vi "F-Truncat-IBRF.vi"() -> ()   [LabVIEW 2014]
doc: "Use this template to build a VI to use as a subVI."
uses:
  <vilib>/vision/NI_Vision_Development_Module.lvlib
panel:
  out "|F(u,v)H(u,v)|":T1(plugin-control)
  out "g(x,y)":T1(plugin-control)
  out "IF(u,v)I":T1(plugin-control)
  out "f(x,y)":T1(plugin-control)
  # ":: MVi Framework V1.0 ::\nAuthor:Gaoke Yang\nEmail: gaoke.yang@yahoo.com\nWeb: www.mvicontrol.com\nCopyright (C) 2015, MVI Technologies All Rights Reserved"
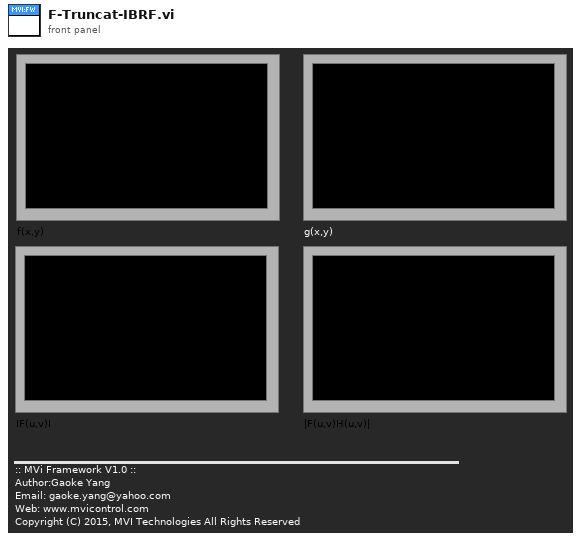
[diagram p1: front panel]
types:
  T1 = typedef "IMAQ Image.ctl" = refnum<image>
  T2 = typedef "Image Type" = u32
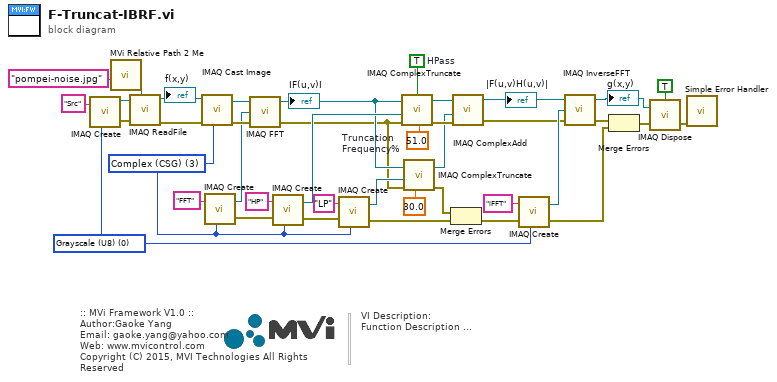
[diagram p0: block diagram]
diagram:
  w20 = sgl 51.0  # Truncation Frequency%
  w21 = TRUE  # HPass
  w19 = T2 0 items=["Grayscale (U8)", "Grayscale (I16)", "Grayscale (SGL)", "Complex (CSG)", "RGB (U32)", "HSL (U32)", "RGB (U64)", "Grayscale (U16)"] ("Image Type")
  w1 = T2 3 items=["Grayscale (U8)", "Grayscale (I16)", "Grayscale (SGL)", "Complex (CSG)", "RGB (U32)", "HSL (U32)", "RGB (U64)", "Grayscale (U16)"] ("Image Type")
  # "VI Description:\nFunction Description ..."
  # ":: MVi Framework V1.0 ::\nAuthor:Gaoke Yang\nEmail: gaoke.yang@yahoo.com\nWeb: www.mvicontrol.com\nCopyright (C) 2015, MVI Technologies All Rights Reserved"
  n1 = call "IMAQ Create"("Image Name"="Src" ("name or relative path"), "Image Type"=w19) -> ("New Image"=w37:T1, "error out"=w36:errorcluster)  [unwired: 2 in, 1 out]
  n2 = call "MVi Relative Path 2 Me.vi"("Relative Path"="pompei-noise.jpg" ("name or relative path")) -> ("Appended Dir"=w33:path)  [unwired: 5 in, 1 out]
  n3 = call "IMAQ ReadFile"("File Path"=w33, "error in (no error)"=w36, "Image"=w37) -> ("error out"=w30:errorcluster, "Image Out"=w29:T1)  [unwired: 4 in, 3 out]
  "f(x,y)" <- w29
  n4 = call "IMAQ Cast Image"("Image Type"=w1, "error in (no error)"=w30, "Image Src"=w29) -> ("error out"=w32:errorcluster, "Image Dst Out"=w28:T1)  [unwired: 7 in]
  n5 = call "IMAQ Create"("Image Name"="FFT" ("name or relative path"), "Image Type"=w1) -> ("New Image"=w27:T1, "error out"=w16:errorcluster)  [unwired: 2 in, 1 out]
  n6 = call "IMAQ FFT"("error in (no error)"=w32, "Image Dst"=w27, "Image Src"=w28) -> ("error out"=w10:errorcluster, "Image Dst Out"=w12:T1)  [unwired: 1 in]
  "IF(u,v)I" <- w12
  n7 = call "IMAQ Create"("Image Name"="HP" ("name or relative path"), "Image Type"=w1, "error in (no error)"=w16) -> ("New Image"=w14:T1, "error out"=w15:errorcluster)  [unwired: 1 in, 1 out]
  n8 = call "IMAQ Create"("Image Name"="LP" ("name or relative path"), "Image Type"=w1, "error in (no error)"=w15) -> ("New Image"=w11:T1, "error out"=w5:errorcluster)  [unwired: 1 in, 1 out]
  n9 = call "IMAQ ComplexTruncate"("error in (no error)"=w10, "Image Dst"=w14, "Truncation Frequency %"=w20, "Image Src"=w12, "Low pass/High pass (Low pass)"=w21) -> ("error out"=w8:errorcluster, "Image Dst Out"=w9:T1)  [unwired: 2 in]
  n10 = call "IMAQ ComplexTruncate"("error in (no error)"=w10, "Image Dst"=w11, "Truncation Frequency %"=sgl 30.0, "Image Src"=w12) -> ("error out"=w6:errorcluster, "Image Dst Out"=w7:T1)  [unwired: 3 in]
  n11 = Merge Errors(w6, w5) -> (w4:errorcluster)
  n12 = call "IMAQ ComplexAdd"("Image Src A"=w9, "Image Src B"=w7, "error in (no error)"=w8) -> ("Image Dst Out"=w2:T1, "error out"=w3:errorcluster)  [unwired: 4 in]
  "|F(u,v)H(u,v)|" <- w2
  n13 = call "IMAQ Create"("Image Name"="iFFT" ("name or relative path"), "Image Type"=w19, "error in (no error)"=w4) -> ("New Image"=w25:T1, "error out"=w22:errorcluster)  [unwired: 1 in, 1 out]
  n14 = call "IMAQ InverseFFT"("error in (no error)"=w3, "Image Dst"=w25, "Image Src"=w2) -> ("error out"=w24:errorcluster, "Image Dst Out"=w23:T1)  [unwired: 1 in]
  "g(x,y)" <- w23
  n15 = Merge Errors(w24, w22) -> (w31:errorcluster)
  n16 = call "IMAQ Dispose"("All Images? (No)"=TRUE, "Image"=w23, "error in (no error)"=w31) -> ("error out"=w38:errorcluster)  [unwired: 3 out]
  n17 = call <vilib>:"Simple Error Handler.vi"("error in (no error)"=w38) -> ()  [unwired: 1 in, 8 out]
